vi "Pre-Close Action.vi"(8 "error in (no error)":errorcluster, 10 "Panel VI":refnum<vi>, 11 "Persistent Position in":refnum<class "Persistent Position.lvclass">) -> (0 "error out":errorcluster)   [LabVIEW 2023, in "Panel Actor.lvlib" / "Panel.lvlib" / "Persistent Position.lvclass"]
doc: "Action to be taken before the panel is closed.\n\n----\nPlease see the following web address for additional documentation and tutorial information:\nhttp://www.mooregoodideas.com/mgi-panel-manager/\n\nAuthor: Derek Trepanier\n\nCopyright (c) 2018, Moore Good Ideas, Inc.\n\nAll rights reserved.\n\nRedistribution and use in source and binary forms, with or without modification, are permitted provided that the following conditions are met:\n\n * Redistributions of source code must retain the above copyright notice, this list of conditions and the following disclaimer.\n * Redistributions in binary form must reproduce the above copyright notice, this list of conditions and the following disclaimer in the documentation and/or other materials provided with the distribution.\n * Neither the name of Moore Good Ideas, Inc. nor the names of its contributors may be used to endorse or promote products derived from this software without specific prior written permission.\n\nTHIS SOFTWARE IS PROVIDED BY THE COPYRIGHT HOLDERS AND CONTRIBUTORS \"AS IS\" AND ANY EXPRESS OR IMPLIED WARRANTIES, INCLUDING, BUT NOT LIMITED TO, THE IMPLIED WARRANTIES OF MERCHANTABILITY AND FITNESS FOR A PARTICULAR PURPOSE ARE DISCLAIMED. IN NO EVENT SHALL THE COPYRIGHT OWNER OR CONTRIBUTORS BE LIABLE FOR ANY DIRECT, INDIRECT, INCIDENTAL, SPECIAL, EXEMPLARY, OR CONSEQUENTIAL DAMAGES (INCLUDING, BUT NOT LIMITED TO, PROCUREMENT OF SUBSTITUTE GOODS OR SERVICES; LOSS OF USE, DATA, OR PROFITS; OR BUSINESS INTERRUPTION) HOWEVER CAUSED AND ON ANY THEORY OF LIABILITY, WHETHER IN CONTRACT, STRICT LIABILITY, OR TORT (INCLUDING NEGLIGENCE OR OTHERWISE) ARISING IN ANY WAY OUT OF THE USE OF THIS SOFTWARE, EVEN IF ADVISED OF THE POSSIBILITY OF SUCH DAMAGE."
uses:
  Persistent Position.lvclass
  Persistent Position.lvclass/Persistent Position.ctl
  <vilib>/Utility/config.llb/Write Key (String).vi
  <vilib>/Utility/config.llb/NI_LVConfig.lvlib
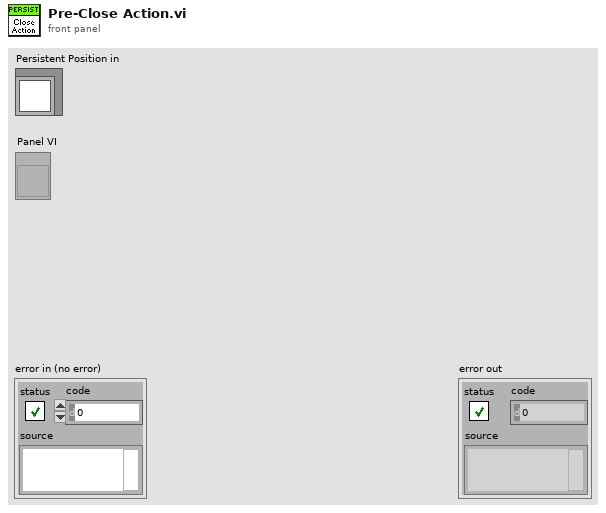
[diagram p1: front panel]
types:
  T1 = enum32{"Invalid", "Standard", "Closed", "Hidden", "Minimized", "Maximized"}
  T2 = typedef "LVRectTypeDef.ctl" = cluster{"Left":i16, "Top":i16, "Right":i16, "Bottom":i16}
  T3 = typedef "NI_LVConfig.lvlib/Config Data RefNum.ctl" = refnum<k1>
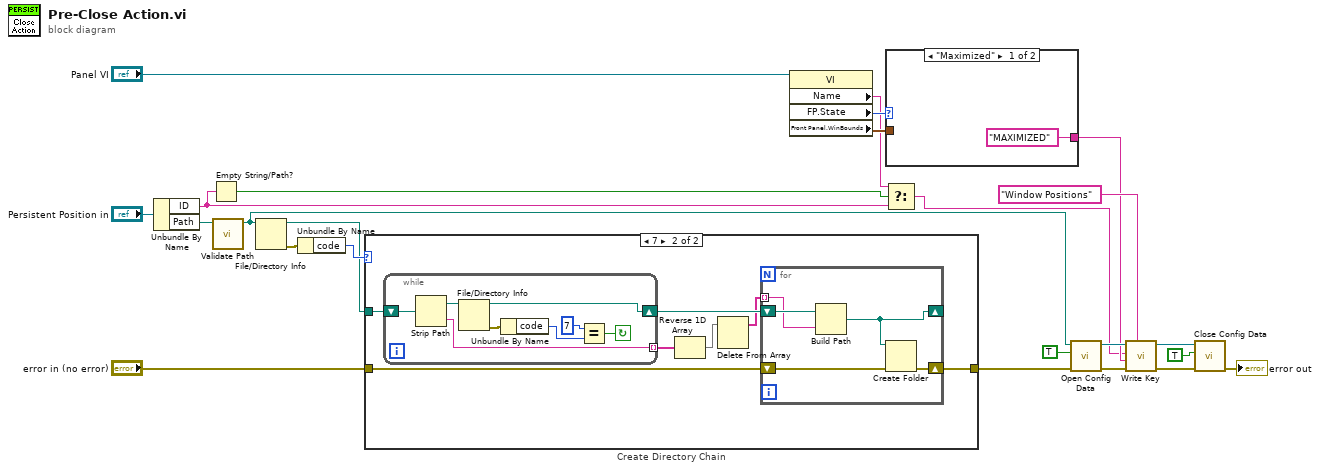
[diagram p0: block diagram]
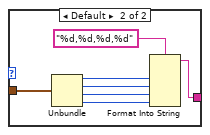
[diagram p2: hidden frame]
diagram:
  n1 = Unbundle By Name("Persistent Position in") -> ("ID"=w2:string, "Path"=w13:path)
  n2 = Empty String/Path?(string/path=w2) -> (empty?=w1:bool)
  n3 = call "Validate Path.vi"("Path in"=w13) -> ("Path out"=w10:path)  [unwired: 10 in]
  n4 = File/Directory Info(path=w10) -> (path out=w22:path, error out=w24:errorcluster)  [unwired: 1 in, 5 out]
  n5 = Unbundle By Name(w24) -> ("code"=w23:i32)
  n6 = case "Create Directory Chain" shown="7" w23 {
    tunnel: "error in (no error)" -> [w25 w30]
    tunnel: [w25 w26] -> w11
    tunnel: w22 -> [_ w29]
    frame Default {
    }
    frame 7 {
      n7 = while {
        shift-right: [w38] -> w31
        shift-left: w29 -> [w45]
        tunnel: [w39] -> w32 mode=indexing
        stop <- w40 continue-if-true
        n8 = Strip Path(path=w45) -> (stripped path=w44:path, name=w39:string)
        n9 = File/Directory Info(path=w44) -> (path out=w38:path, error out=w43:errorcluster)  [unwired: 1 in, 5 out]
        n10 = Unbundle By Name(w43) -> ("code"=w42:i32)
        n11 = Equal?(x=7 ("y"), y=w42) -> (x = y?=w40:bool)
      }
      n12 = Reverse 1D Array(array=w32) -> (reversed array=w28:string[])
      n13 = Delete From Array(array=w28) -> (array with subset deleted=w27:string[])  [unwired: 2 in, 1 out]
      n14 = for {
        shift-right: [w33] -> _
        shift-left: w31 -> [w37]
        tunnel: w27 -> [w36] mode=indexing
        shift-right: [w34] -> w26
        shift-left: w30 -> [w35]
        n15 = Build Path(base path=w37, name or relative path=w36) -> (appended path=w33:path)
        n16 = Create Folder(path (use dialog)=w33, error in=w35) -> (error out=w34:errorcluster)  [unwired: 1 in, 2 out]
      }
    }
  }
  n17 = property class="VI"(reference="Panel VI") -> ("Name"=w4:string, "FP.State"=w7:T1, "Front Panel.WinBounds"=w8:T2)  [unwired: 1 in, 2 out]
  n18 = case shown="\"Maximized\"" w7 {
    tunnel: w8 -> [_ w53]
    tunnel: ["MAXIMIZED" ("default value") w47] -> w5
    frame "Maximized" {
    }
    frame Default {
      n19 = Unbundle(w53) -> ("Left"=w52:i16, "Top"=w51:i16, "Right"=w50:i16, "Bottom"=w49:i16)
      n20 = Format Into String(format string="%d,%d,%d,%d", w52, w51, w50, w49) -> (resulting string=w47:string)  [unwired: 2 in, 1 out]
    }
  }
  n21 = Select(t=w4, s=w1, f=w2) -> (s? t:f=w3:string)
  n22 = call <vilib>:"Open Config Data.vi"("error in (no error)"=w11, "create file if necessary (T)"=TRUE, "configuration file path"=w10) -> ("error out"=w21:errorcluster, "refnum"=w20:T3)  [unwired: 6 in, 1 out]
  n23 = call-poly <vilib>:"Write Key.vi"("section"="Window Positions", "error in (no error)"=w21, "value"=w5, "key"=w3, "refnum"=w20) -> ("error out"=w18:errorcluster, "refnum out"=w19:T3)  [unwired: 4 in, 1 out]
  n24 = call <vilib>:"Close Config Data.vi"("error in (no error)"=w18, "write file if changed (T)"=TRUE, "refnum"=w19) -> ("error out"=→"error out":errorcluster)  [unwired: 7 in, 1 out]
